vi "Layout.vi"(8 "error in (no error)":errorcluster, 11 "FSM in":refnum<class "FSM.Graph.lvclass">) -> (0 "error out":errorcluster, 3 "FSM out":refnum<class "FSM.Graph.lvclass">)   [LabVIEW 2015, in "FSM.Graph.lvclass"]
uses:
  FSM.Graph.lvclass
  FSM.Graph.lvclass/FSM.Graph.ctl
  FSM.Node/FSM.Node.lvclass
  FSM.Edge/FSM.Edge.lvclass
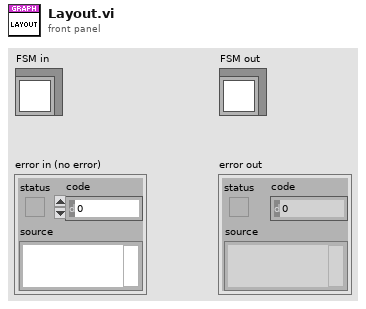
[diagram p1: front panel]
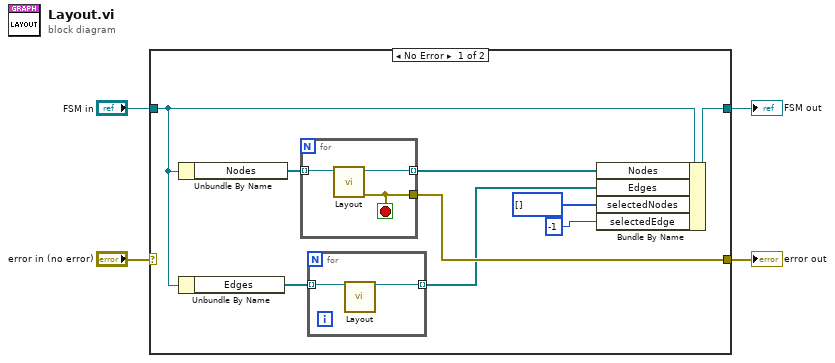
[diagram p0: block diagram]
diagram:
  n1 = case shown="No Error" "error in (no error)" {
    selector: "error in (no error)" -> [_ w20]
    tunnel: [w12 w20] -> w3
    tunnel: [w11 w19] -> w1
    tunnel: "FSM in" -> [w7 w19]
    frame No Error {
      n2 = Unbundle By Name(w7) -> ("Nodes"=w13:refnum<class "FSM.Node.lvclass">[])
      n3 = Unbundle By Name(w7) -> ("Edges"=w6:refnum<class "FSM.Edge.lvclass">[])
      n4 = for {
        tunnel: w13 -> [w18] mode=indexing
        tunnel: [w16] -> w12
        tunnel: [w17] -> w10 mode=indexing
        stop <- w16 stop-if-true
        n5 = call "Layout.vi"("FSM in"=w18) -> ("error out"=w16:errorcluster, "FSM out"=w17:refnum<class "FSM.Node.lvclass">)  [unwired: 9 in]
      }
      n6 = for {
        tunnel: w6 -> [w15] mode=indexing
        tunnel: [w14] -> w5 mode=indexing
        n7 = call "Layout.vi"("FSM.Edge In"=w15) -> ("FSM.Edge Out"=w14:refnum<class "FSM.Edge.lvclass">)  [unwired: 14 in]
      }
      n8 = Bundle By Name(cluster=w7, "Nodes"=w10, "Edges"=w5, "selectedNodes"=i32[] [], "selectedEdge"=-1) -> (w11:refnum<class "FSM.Graph.lvclass">)
    }
    frame Error {
    }
  }
  "error out" <- w3
  "FSM out" <- w1
